vi "niRFUtil MASMT Util Get 2D CDB Type.vi"(1 "2D CDB Array in":cdb[][](array[numeric])) -> (0 "2D CDB Array out":cdb[][](array[numeric]))   [LabVIEW 2015, in "niRFUtil.lvlib"]
uses:
  niRFUtil.lvlib
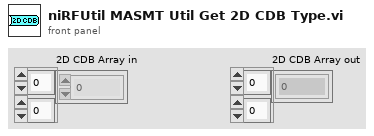
[diagram p1: front panel]
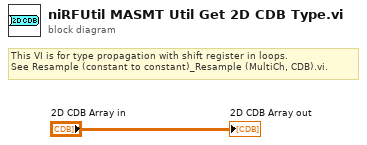
[diagram p0: block diagram]
diagram:
  # "This VI is for type propagation with shift register in loops.\nSee Resample (constant to constant)_Resample (MultiCh, CDB).vi."
  "2D CDB Array out" <- "2D CDB Array in"
